vi "ECU Selector64.vi"(6 "ECU TYPE":u16(ring) items=["LSMD", "LSMP", "LSMRL", "LSMRR"]) -> (0 "ID Response":string, 1 "Puerto DAQ":i32, 2 "Numeric Request":i32=416962034 format="%x", 3 "ID Request":string, 4 "frame":refnum<k21>="Escritura_Driver\nElatch Database")   [LabVIEW 2023]
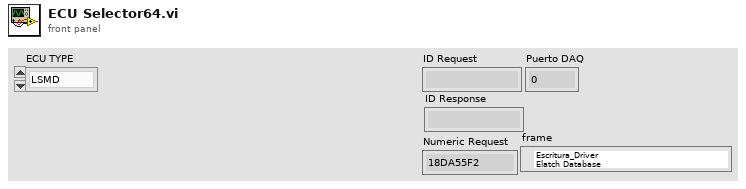
[diagram p1: front panel]
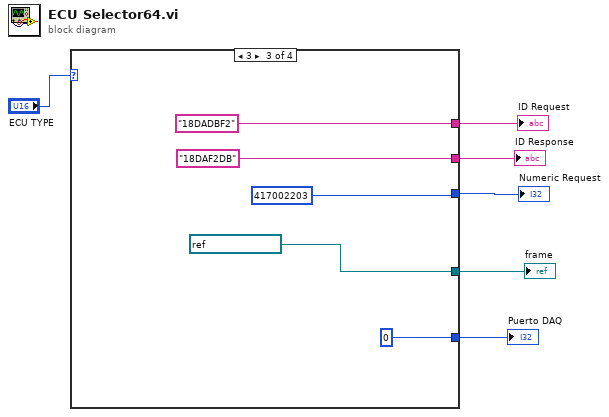
[diagram p0: block diagram]
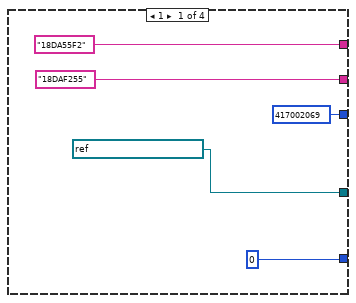
[diagram p2: hidden frame]
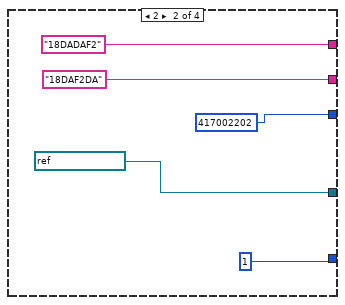
[diagram p3: hidden frame]
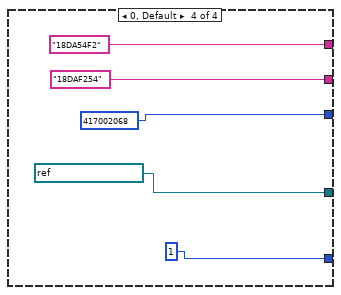
[diagram p4: hidden frame]
diagram:
  n1 = case shown="3" "ECU TYPE" {
    tunnel: ["18DA55F2" "18DADAF2" "18DADBF2" "18DA54F2"] -> w5
    tunnel: ["18DAF255" "18DAF2DA" "18DAF2DB" "18DAF254"] -> w4
    tunnel: [417002069 417002202 417002203 417002068] -> w3
    tunnel: [refnum<k21> "Escritura_Passenger\nElatch Database" ("frame") refnum<k21> "Escritura_RL\nElatch Database" ("frame") refnum<k21> "Escritura_RR\nElatch Database" ("frame") refnum<k21> "Escritura_Driver\nElatch Database" ("frame")] -> w2
    tunnel: [0 1 0 1] -> w1
    frame 1 {
    }
    frame 2 {
    }
    frame 3 {
    }
    frame 0, Default {
    }
  }
  "ID Request" <- w5
  "ID Response" <- w4
  "Numeric Request" <- w3
  "frame" <- w2
  "Puerto DAQ" <- w1
